vi "LVClass_CorrectionDataManager SaveInteractrionMatrix.vi"(0 "CorrectionDataManager in":refnum<class "CorrectionDataManager.lvclass">, 7 "Interaction Matrix file path":path, 9 "comment":string, 11 "error in (no error)":errorcluster) -> (4 "CorrectionDataManager out":refnum<class "CorrectionDataManager.lvclass">, 15 "error out":errorcluster)   [LabVIEW 2020, in "CorrectionDataManager.lvclass"]
doc: "Dumps CorrDataManager data to file.\n\n<B>corrdata_managerIn</B> : CorrDataManager object.\n<B>corrdata_managerOut</B> : CorrDataManager object.\n<B>backup_file_path</B> : Absolute path to CorrDataManager backup file.\n<B>comment</B> : User-defined comment to write to backup file."
uses:
  CorrectionDataManager.lvclass
  CorrectionDataManager.lvclass/CorrectionDataManager.ctl
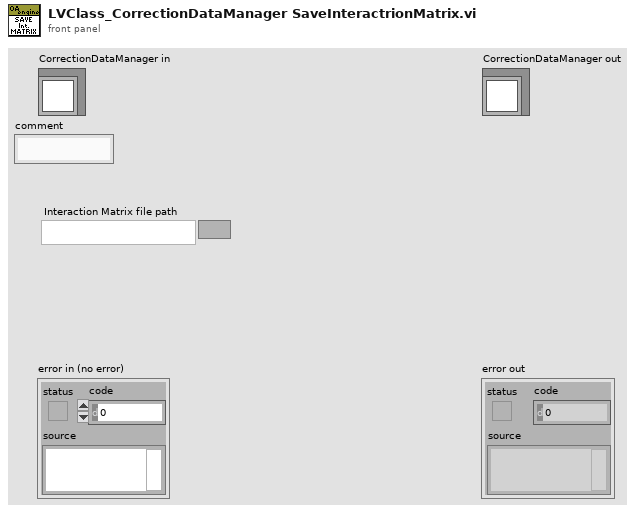
[diagram p1: front panel]
types:
  T1 = typedef "ClassID.ctl" = i64
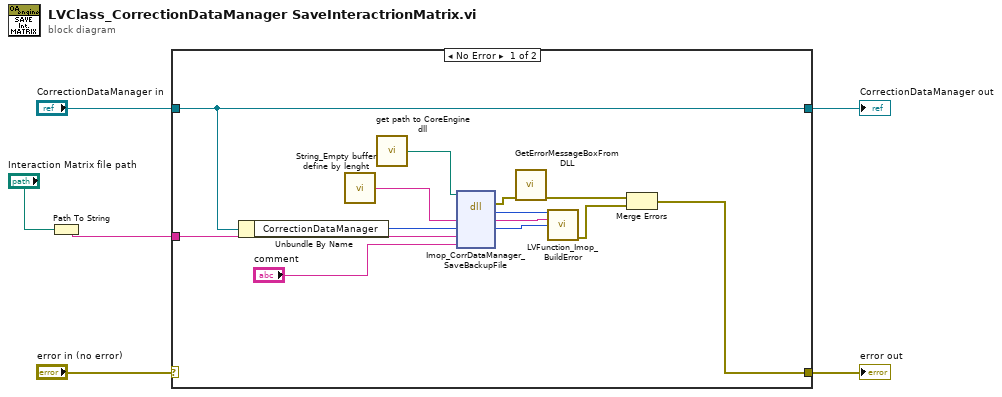
[diagram p0: block diagram]
diagram:
  n1 = Path To String(path="Interaction Matrix file path") -> (string=w1:string)
  n2 = case shown="No Error" "error in (no error)" {
    selector: "error in (no error)" -> [_ w21]
    tunnel: [w11 w21] -> w3
    tunnel: [w12 w20] -> w6
    tunnel: "CorrectionDataManager in" -> [w12 w20]
    tunnel: w1 -> [w9 _]
    frame No Error {
      n3 = Unbundle By Name(w12) -> ("CorrectionDataManager"=w10:T1)
      n4 = call "String_Empty buffer define by lenght.vi"() -> ("Empty buffer"=w17:string)  [unwired: 1 in]
      n5 = call "get path to CoreEngine dll.vi"() -> ("path to wavekit library"=w16:path)  [unwired: 14 in, 1 out]
      n6 = dll-call lib="D:/soft/HASO_v3/SVN_trunk/ImOpCoreEngine4_LV2011/DLLs/c_interface_vc100.dll" fn="Imop_CorrDataManager_SaveBackupFile"(path in=w16, "message"=w17, "WavefrontCorrection"=w10, "backup_file_path"=w9, "comment"="comment") -> (error out=w15:errorcluster, "return type"=w19:i32, "message"=w18:string, "WavefrontCorrection"=w7:i64)  [unwired: 4 in, 1 out]
      n7 = call "GetErrorMessageBoxFromDLL.vi"("error IN"=w15) -> ("error OUT"=w14:errorcluster)  [unwired: 10 in]
      n8 = call "LVFunction_Imop_BuildError.vi"("code"=w19, "String to Prepend to source (\"\")"=w18, "Adresse"=w7) -> ("error out"=w13:errorcluster)  [unwired: 12 in]
      n9 = Merge Errors(w14, w13) -> (w11:errorcluster)
    }
    frame Error {
    }
  }
  "error out" <- w3
  "CorrectionDataManager out" <- w6
